vi "_Read.vi"(8 "error in (no error)":errorcluster, 11 "Fluke Multimeter in":refnum<class "Fluke Multimeter.lvclass">) -> (0 "error out":errorcluster, 2 "4 Data Points":dbl[](array[numeric]), 3 "Fluke Multimeter out":refnum<class "Fluke Multimeter.lvclass">)   [LabVIEW 2009, in "Fluke Multimeter.lvclass"]
doc: "(Protected, Dynamic) Perform a measurement and return up to four channels of data. Outsiders should not call this method, but instead the public \"Read Data.vi\"."
uses:
  Fluke Multimeter.lvclass
  Utility Classes/Readable/Readable.lvclass
  Fluke 8840/Fluke 8840.lvlib
panel:
  in  "function (0:volts DC)":u16(ring) items=["volts DC", "volts AC", "2-wire k.ohms", "4-wire k.ohms", "mA DC", "mA AC"]
  in  "range (0:auto)":u16(ring) items=["autorange", "200mV, 200 ohms", "2V, 2 kohms", "20V, 20 kohms", "200V, 200 kohms", "1000Vdc, 700 Vac, 2 Mohms", "20 Mohms"]
  in  "rate (0:slow)":u16(ring) items=["slow", "medium", "fast"]
  in  "trigger mode (0:internal)":u16(ring) items=["internal - continuous trigger", "external - rear panel trigger with delay", "external - bus trigger with delay", "external - rear panel trigger", "external - bus trigger"]
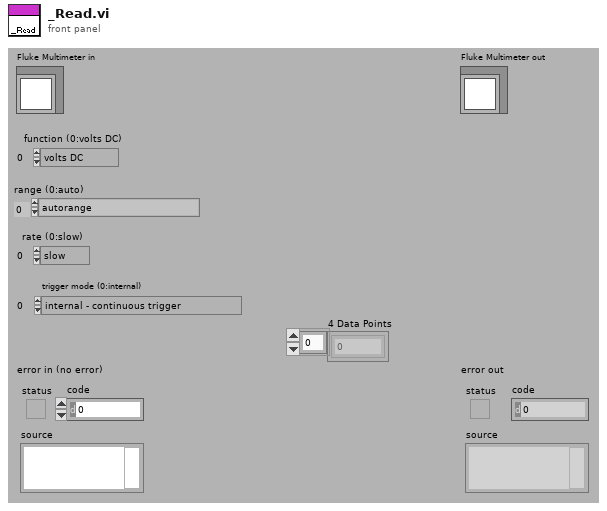
[diagram p1: front panel]
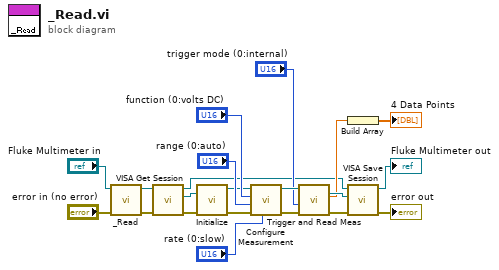
[diagram p0: block diagram]
diagram:
  n1 = call-parent "_Read.vi"("error in (no error)"="error in (no error)", "Readable in"="Fluke Multimeter in") -> ("error out"=w3:errorcluster, "Readable out"=w10:refnum<class "Fluke Multimeter.lvclass">)  [unwired: 8 out]
  n2 = call-dynamic "VISA Get Session.vi"("error in (no error)"=w3, "Instrument.lvclass in"=w10) -> ("error out"=w2:errorcluster, "VISA Resource Name"=w11:refnum<visa-resource-name>, "Instrument.lvclass out"=w4:refnum<class "Fluke Multimeter.lvclass">)  [unwired: 7 out]
  n3 = call "Initialize.vi"("error in (no error)"=w2, "VISA resource name"=w11) -> ("error out"=w15:errorcluster, "VISA resource name out"=w16:refnum<visa-resource-name>)  [unwired: 1 in, 7 out]
  n4 = call "Configure Measurement.vi"("rate (0:slow)"="rate (0:slow)", "error in (no error)"=w15, "range (0:auto)"="range (0:auto)", "function (0:volts DC)"="function (0:volts DC)", "VISA resource name"=w16) -> ("error out"=w13:errorcluster, "VISA resource name out"=w14:refnum<visa-resource-name>)  [unwired: 5 out]
  n5 = call "Trigger and Read Meas.vi"("error in (no error)"=w13, "trigger mode (0:internal)"="trigger mode (0:internal)", "VISA resource name"=w14) -> ("error out"=w7:errorcluster, "measurement"=w6:dbl, "VISA resource name out"=w8:refnum<visa-resource-name>)  [unwired: 6 out]
  n6 = Build Array(w6) -> (→"4 Data Points":dbl[])
  n7 = call-dynamic "VISA Save Session.vi"("error in (no error)"=w7, "VISA Resource Name"=w8, "Instrument.lvclass in"=w4) -> ("error out"=→"error out":errorcluster, "Instrument.lvclass out"=→"Fluke Multimeter out":refnum<class "Fluke Multimeter.lvclass">)  [unwired: 7 out]
